vi "GetCurrentCommand.vi"(8 "error in (no error)":errorcluster, 11 "PathTokenizer in":refnum<class "PathTokenizer.lvclass">) -> (0 "error out":errorcluster, 1 "Index":i32, 2 "Character":string, 3 "PathTokenizer out":refnum<class "PathTokenizer.lvclass">, 4 "Found?":bool)   [LabVIEW 2020]
uses:
  PathTokenizer.lvclass
  PathTokenizer.lvclass/PathTokenizer.ctl
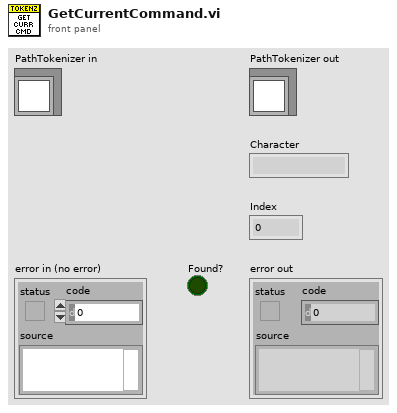
[diagram p1: front panel]
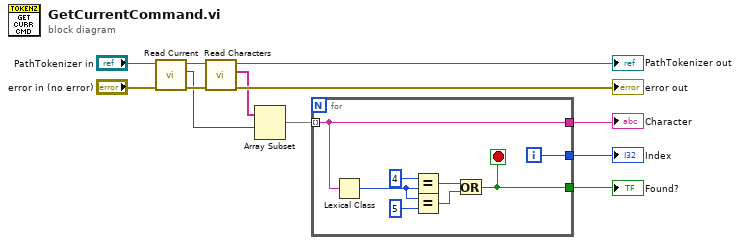
[diagram p0: block diagram]
diagram:
  n1 = call "Read Current.vi"("error in (no error)"="error in (no error)", "PathTokenizer in"="PathTokenizer in") -> ("error out"=w12:errorcluster, "Current"=w1:i32, "PathTokenizer out"=w4:refnum<class "PathTokenizer.lvclass">)  [unwired: 7 in]
  n2 = call "Read Characters.vi"("error in (no error)"=w12, "PathTokenizer in"=w4) -> ("error out"=→"error out":errorcluster, "Characters"=w3:string[], "PathTokenizer out"=→"PathTokenizer out":refnum<class "PathTokenizer.lvclass">)  [unwired: 7 in]
  n3 = Array Subset(array=w3, index=w1) -> (w2:string[])  [unwired: 1 in]
  n4 = for {
    tunnel: w2 -> [w14] mode=indexing
    tunnel: [w15] -> w7
    tunnel: [w14] -> w6
    tunnel: [w13] -> w5
    i -> [w15]
    stop <- w13 stop-if-true
    n5 = Lexical Class(1:w14) -> (0:w19:i16)
    n6 = Equal?(x=i16 4, y=w19) -> (x = y?=w17:bool)
    n7 = Equal?(x=w19, y=i16 5) -> (x = y?=w16:bool)
    n8 = Or(x=w17, y=w16) -> (x .or. y?=w13:bool)
  }
  "Index" <- w7
  "Character" <- w6
  "Found?" <- w5
